vi "Bit-array To Byte-array.vi"(1 "bit array":bool[][](array[boolean])) -> (0 "byte array":u8[](array[numeric]))   [LabVIEW 2014]
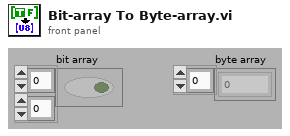
[diagram p1: front panel]
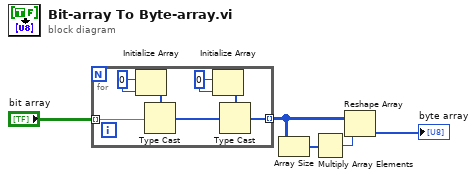
[diagram p0: block diagram]
diagram:
  n1 = for {
    tunnel: [w9] -> w3 mode=indexing
    tunnel: "bit array" -> [w6] mode=indexing
    w8 = u8 0
    w11 = i16 0
    n2 = Initialize Array(w11, w11) -> (w12:i16[])
    n3 = Type Cast(type=w12, x=w6) -> (*(type *) &x=w10:i16[])
    n4 = Initialize Array(w8, w8) -> (w7:u8[])
    n5 = Type Cast(type=w7, x=w10) -> (*(type *) &x=w9:u8[])
  }
  n6 = Array Size(array=w3) -> (size(s)=w1:i32[])
  n7 = Multiply Array Elements(1:w1) -> (0:w2:i32)
  n8 = Reshape Array(w3, w2) -> (→"byte array":u8[])
